vi "Notify Launcher.vi"(8 "error in (no error)":errorcluster, 9 "milliseconds to wait":u32, 10 "Notification":string, 11 "Application Controller in":refnum<class "Application Controller.lvclass">) -> (0 "error out":errorcluster, 3 "Application Controller out":refnum<class "Application Controller.lvclass">)   [LabVIEW 2019, in "Application Controller.lvclass"]
uses:
  Application Controller.lvclass
  Application Controller.lvclass/Application Controller.ctl
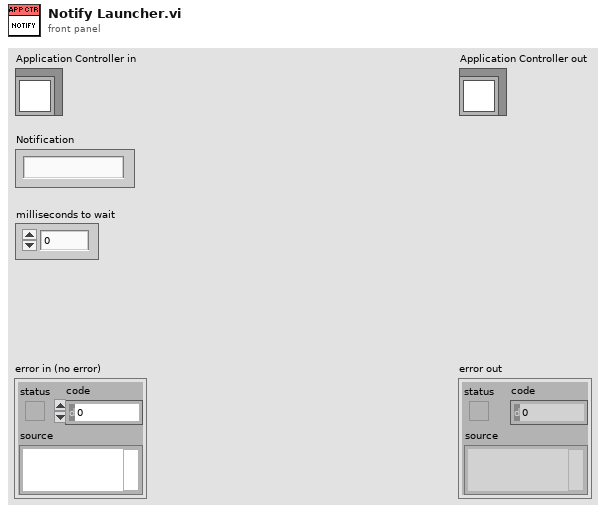
[diagram p1: front panel]
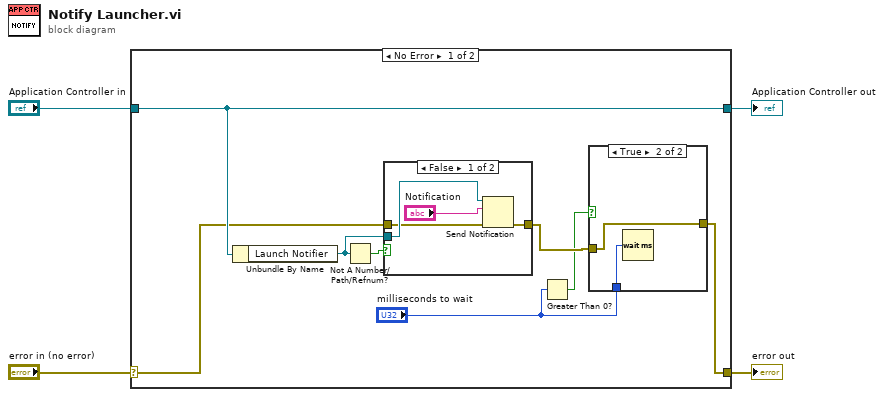
[diagram p0: block diagram]
diagram:
  n1 = case shown="No Error" "error in (no error)" {
    selector: "error in (no error)" -> [w9 w22]
    tunnel: [w7 w22] -> w3
    tunnel: [w10 w21] -> w1
    tunnel: "Application Controller in" -> [w10 w21]
    frame No Error {
      n2 = Unbundle By Name(w10) -> ("Launch Notifier"=w12:refnum<notifier>)
      n3 = Not A Number/Path/Refnum?(number/path/refnum=w12) -> (NaN/Path/Refnum?=w11:bool)
      n4 = case shown="False" w11 {
        tunnel: w12 -> [w18 _]
        tunnel: w9 -> [w17 w20]
        tunnel: [w16 w20] -> w8
        frame False {
          n5 = Send Notification(notification="Notification", notifier=w18, error in (no error)=w17) -> (error out=w16:errorcluster)  [unwired: 1 out]
        }
        frame True {
        }
      }
      n6 = Greater Than 0?(x="milliseconds to wait") -> (x > 0?=w5:bool)
      n7 = case shown="True" w5 {
        tunnel: "milliseconds to wait" -> [_ w15]
        tunnel: w8 -> [w13 w14]
        tunnel: [w13 w14] -> w7
        frame False {
        }
        frame True {
          n8 = Wait (ms)(milliseconds to wait=w15) -> ()  [unwired: 1 out]
        }
      }
    }
    frame Error {
    }
  }
  "error out" <- w3
  "Application Controller out" <- w1
